vi "mecanum_get_commands.vi"(11 "Joysticks":T3) -> (3 "Mecanum":T1)   [LabVIEW 2012]
uses:
  <vilib>/Rock Robotics/WPI/Joystick/WPI_JoystickButtonState.ctl
  mecanum_control.ctl
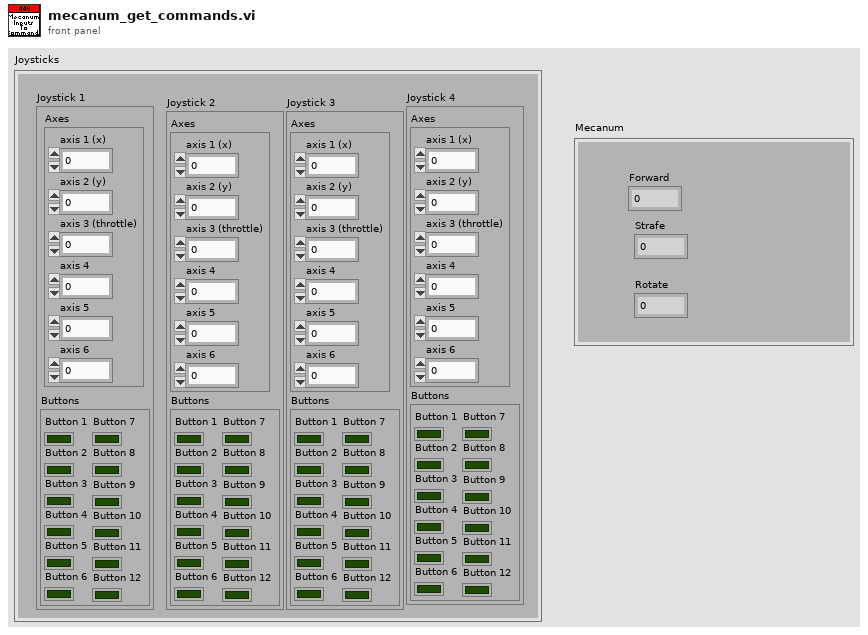
[diagram p1: front panel]
types:
  T1 = typedef "mecanum_control.ctl" = cluster{"Forward":dbl, "Strafe":dbl, "Rotate":dbl}
  T2 = typedef "WPI_JoystickButtonState.ctl" = cluster{"Button 1":bool, "Button 2":bool, "Button 3":bool, "Button 4":bool, "Button 5":bool, "Button 6":bool, "Button 7":bool, "Button 8":bool, "Button 9":bool, "Button 10":bool, "Button 11":bool, "Button 12":bool}
  T3 = cluster{"Joystick 1":cluster{"Axes":cluster{"axis 1 (x)":dbl, "axis 2 (y)":dbl, "axis 3 (throttle)":dbl, "axis 4":dbl, "axis 5":dbl, "axis 6":dbl}, "Buttons":T2}, "Joystick 2":cluster{"Axes":cluster{"axis 1 (x)":dbl, "axis 2 (y)":dbl, "axis 3 (throttle)":dbl, "axis 4":dbl, "axis 5":dbl, "axis 6":dbl}, "Buttons":T2}, "Joystick 3":cluster{"Axes":cluster{"axis 1 (x)":dbl, "axis 2 (y)":dbl, "axis 3 (throttle)":dbl, "axis 4":dbl, "axis 5":dbl, "axis 6":dbl}, "Buttons":T2}, "Joystick 4":cluster{"Axes":cluster{"axis 1 (x)":dbl, "axis 2 (y)":dbl, "axis 3 (throttle)":dbl, "axis 4":dbl, "axis 5":dbl, "axis 6":dbl}, "Buttons":T2}}
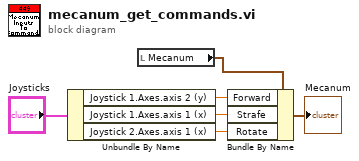
[diagram p0: block diagram]
diagram:
  n1 = Unbundle By Name("Joysticks") -> ("Joystick 1.Axes.axis 2 (y)"=w2:dbl, "Joystick 1.Axes.axis 1 (x)"=w1:dbl, "Joystick 2.Axes.axis 1 (x)"=w3:dbl)
  n2 = local read "Mecanum"() -> (w4:T1)
  n3 = Bundle By Name(cluster=w4, "Forward"=w2, "Strafe"=w1, "Rotate"=w3) -> (→"Mecanum":T1)
